vi "channel operation tests.vi"() -> ()   [LabVIEW 2013, in "tdms logger tests.lvlib"]
uses:
  tdms logger tests.lvlib
  configuration/TDMS datalogger configuration.lvclass
panel:
  out "channels match":bool
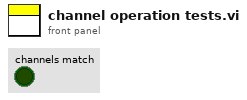
[diagram p1: front panel]
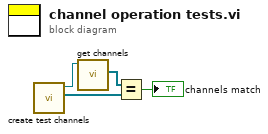
[diagram p0: block diagram]
diagram:
  n1 = call "create test channels.vi"() -> ("chans"=w1:refnum<class "TBM channel.lvclass">[], "TDMS datalogger configuration out"=w2:refnum<class "TDMS datalogger configuration.lvclass">)  [unwired: 8 in, 2 out]
  n2 = call-dynamic "get channels.vi"("module configuration in"=w2) -> ("channels"=w4:refnum<class "TBM channel.lvclass">[])  [unwired: 9 in, 1 out]
  n3 = Equal?(x=w4, y=w1) -> (x = y?=→"channels match":bool)
